vi "Drive Controller.vi"(8 "error in":errorcluster) -> ()   [LabVIEW 2019]
doc: "This VI executes continuously carrying out the current operation and responding to updates or new operation requests. It will often contain the timing or control code that is difficult to place directly in TeleOp. This VI generally opens all sensors and motors and isolates the rest of the robot code from knowing implementation details of how the operations are carried out."
uses:
  <vilib>/Rock Robotics/WPI/Framework/Completion Status.ctl
  Drive Setpoints.ctl
  Drive Operations.ctl
  <vilib>/Rock Robotics/WPI/ThirdParty/REV Robotics/SPARK MAX/Typedef/Spark MAX Control Type.ctl
panel:
  out "L v 2":dbl(graph)
  out "L setpoint 2":dbl(graph)
  out "R setpoint 2":dbl(graph)
  out "R v":dbl(graph)
  out "L v":dbl(graph)
  out "L setpoint":dbl(graph)
  out "R setpoint":dbl(graph)
  out "Immediate graph":dbl(graph)
  in  "Interactive Values":T1
  in  "Buttons":cluster{"Execute Cmd":bool, "Abort Cmd":bool}
  out "Command Timing":cluster{"Start Time (ms)":u32, "Iterations":i32}
  out "Status":T3
  out "Current\nCmd":string
  # "Tip: The graph shows the motor setpoints. It may also be helpful to observe inputs and sensor values.\nYou may also want to display tuning or debugging controls."
  # "Interactive Command: You may fill in the settings for a command\nand schedule it with the Execute button. You can observe and abort\nany command while fine tuning the code for the controller."
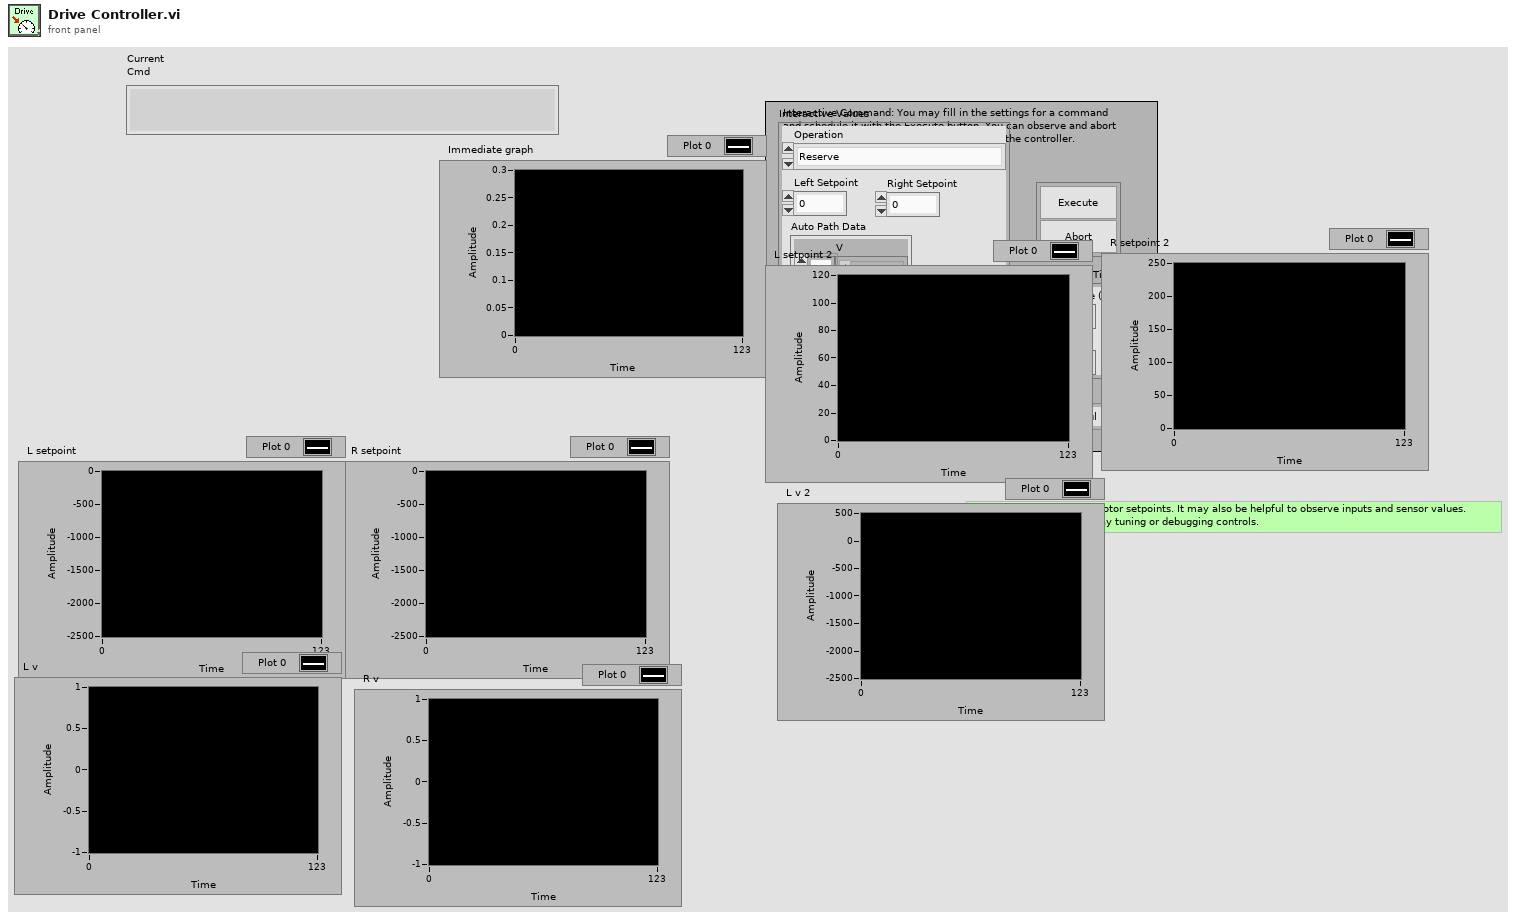
[diagram p1: front panel]
types:
  T1 = typedef "Drive Setpoints.ctl" = cluster{"Operation":T2, "Left Setpoint":dbl, "Right Setpoint":dbl, "Auto Path Data":cluster{"V":dbl[], "Theta":dbl[], "Sample Period":dbl}}
  T2 = typedef "Drive Operations.ctl" = enum16{"Reserve", "Read Current", "Immediate", "Drive for Time", "Drive for Distance", "Play Path", "Play Path Rev"}
  T3 = typedef "Completion Status.ctl" = enum16{"Successful", "Aborted", "Incomplete"}
  T4 = typedef "WPI_MotorControlDeviceRef.ctl" = cluster{"DeviceStatus":errorcluster, "Type":T5, "PWM":cluster{"PWM Channel":T6, "DeadBand":T7}, "CAN":cluster{"Device Number":u8, "SetOutput VI Ref":variant, "GetOutput VI Ref":variant, "Enable VI Ref":variant, "Disable VI Ref":variant, "Data":variant}, "Invert":bool, "DIO PWM":cluster{"PWM \"Enable\" Channel":T6, "DIOChannel":T8, "PWM Rate":dbl}}
  T5 = typedef "WPI_MotorControlType.ctl" = enum16{"PWM", "CAN", "DIO PWM"}
  T6 = typedef "FPGA_DIOPWMChannel.ctl" = enum8{"PWM 0", "PWM 1", "PWM 2", "PWM 3", "PWM 4", "PWM 5", "PWM 6", "PWM 7", "PWM 8", "PWM 9", "PWM MXP 0", "PWM MXP 1", "PWM MXP 2", "PWM MXP 3", "PWM MXP 4", "PWM MXP 5", "PWM MXP 6", "PWM MXP 7", "PWM MXP 8", "PWM MXP 9", "Invalid"}
  T7 = typedef "WPI_PWMDeadband.ctl" = cluster{"Name":string, "maxPositivePwm":i32, "minPositivePwm":i32, "centerPwm":i32, "maxNegativePwm":i32, "minNegativePwm":i32, "angularRange":u16}
  T8 = typedef "FPGA_DIOChannel.ctl" = enum8{"DIO 0", "DIO 1", "DIO 2", "DIO 3", "DIO 4", "DIO 5", "DIO 6", "DIO 7", "DIO 8", "DIO 9", "DIO MXP 0", "DIO MXP 1", "DIO MXP 2", "DIO MXP 3", "DIO MXP 4", "DIO MXP 5", "DIO MXP 6", "DIO MXP 7", "DIO MXP 8", "DIO MXP 9", "DIO MXP 10", "DIO MXP 11", "DIO MXP 12", "DIO MXP 13", "DIO MXP 14", "DIO MXP 15", "SPI Port CS1", "SPI Port CS2", "SPI Port CS3", "SPI Port MISO", "SPI Port MOSI", "Invalid"}
  T9 = typedef "Command Status Info.ctl" = cluster{"Name":string, "Status":T3, "notifier out":T10}
  T10 = typedef "Completion Notifier.ctl" = refnum<notifier>
  T11 = cluster{"SubSystem Data":T1, cluster{"Start Time (ms)":u32, "Iterations":i32}, cluster{"Command Info":T9, "Description":string, "Default Command":T1, "queue out":refnum<queue>, "Subsystem Name":string}}
  T12 = typedef "Spark MAX Control Type.ctl" = enum16{"Percent VBus", "Voltage", "Velocity", "Position", "Smart Motion", "Current", "Smart Velocity"}
  T13 = cluster{"V":dbl[], "Theta":dbl[], "Sample Period":dbl}
  T14 = cluster{"SubSystem Data":T1, cluster{"Start Time (ms)":u32, "Iterations":i32}, "Default Command Arguments":cluster{"Command Info":T9, "Description":string, "Default Command":T1, "queue out":refnum<queue>, "Subsystem Name":string}}
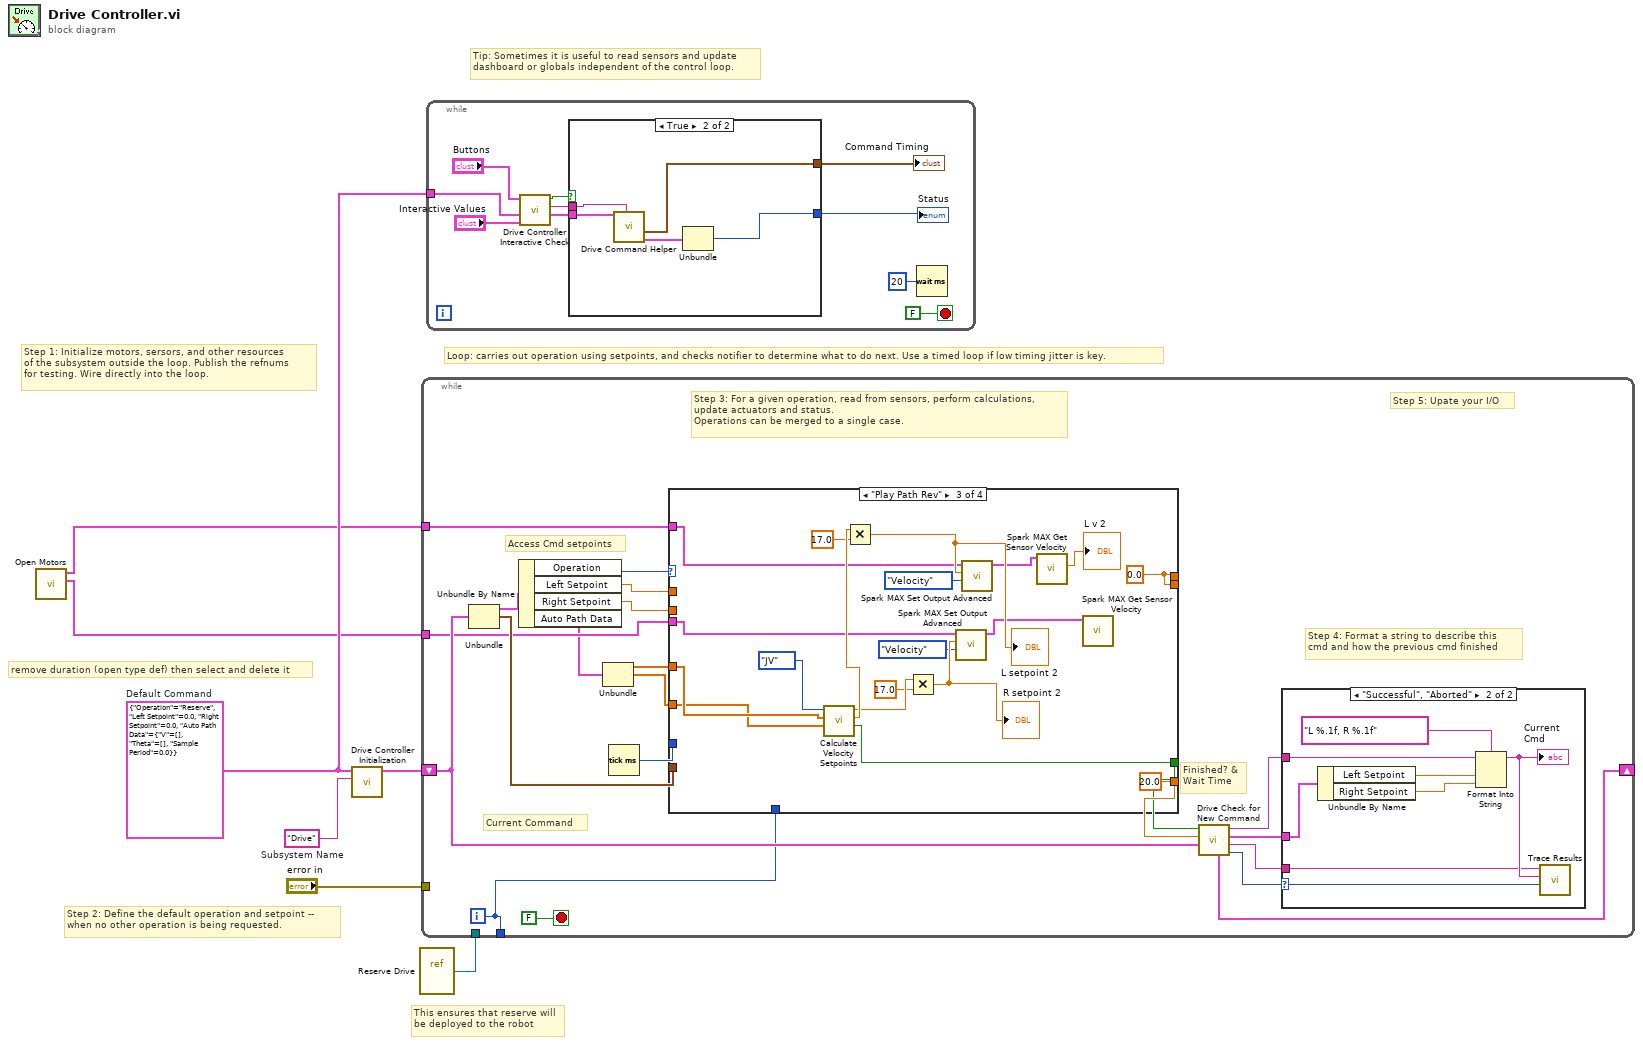
[diagram p0: block diagram]
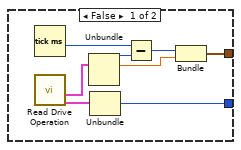
[diagram p2: hidden frame]
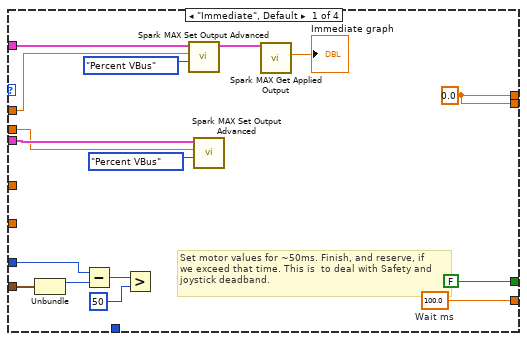
[diagram p4: hidden frame]
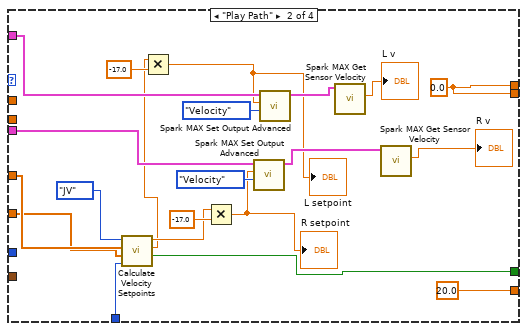
[diagram p5: hidden frame]
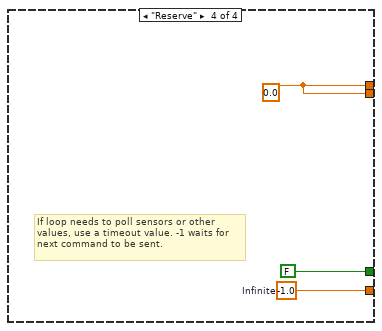
[diagram p6: hidden frame]
diagram:
  w3 = T1 {"Operation"=enum."Reserve", "Left Setpoint"=0.0, "Right Setpoint"=0.0, "Auto Path Data"={"V"=[], "Theta"=[], "Sample Period"=0.0}}  # Default Command
  w7 = "Drive"  # Subsystem Name
  # "remove duration (open type def) then select and delete it"
  # "This ensures that reserve will\nbe deployed to the robot"
  # "Tip: Sometimes it is useful to read sensors and update\ndashboard or globals independent of the control loop."
  # "Step 2: Define the default operation and setpoint --\nwhen no other operation is being requested."
  # "Step 1: Initialize motors, sersors, and other resources\nof the subsystem outside the loop. Publish the refnums\nfor testing. Wire directly into the loop."
  # "Loop: carries out operation using setpoints, and checks notifier to determine what to do next. Use a timed loop if low timing jitter is key."
  n1 = call "Open Motors.vi"() -> ("Right"=w1:T4, "Left"=w2:T4)  [unwired: 10 in]
  n2 = call "Drive Controller Initialization.vi"("Subsystem Name"=w7, "Default Command"=w3) -> ("Current Command"=w5:T11)  [unwired: 9 in]
  n3 = vi-ref "Reserve Drive.vi"() -> (w4:refnum<vi>)
  n4 = while {
    shift-right: [w21] -> _
    shift-left: w5 -> [w14]
    tunnel: [w8] -> _
    tunnel: "error in" -> [_]
    tunnel: w4 -> [_]
    tunnel: w2 -> [w13]
    tunnel: w1 -> [w12]
    i -> [w8]
    stop <- FALSE stop-if-true
    # "Step 5: Upate your I/O"
    # "Step 4: Format a string to describe this\ncmd and how the previous cmd finished"
    # "Current Command"
    # "Access Cmd setpoints"
    # "Finished? &\nWait Time"
    # "Step 3: For a given operation, read from sensors, perform calculations,\nupdate actuators and status.\nOperations can be merged to a single case."
    n5 = Unbundle(w14) -> ("SubSystem Data"=w27:T1, w15:cluster{"Start Time (ms)":u32, "Iterations":i32})  [unwired: 1 out]
    n6 = Unbundle By Name(w27) -> ("Operation"=w26:T2, "Left Setpoint"=w25:dbl, "Right Setpoint"=w24:dbl, "Auto Path Data"=w11:T13)
    n7 = Unbundle(w11) -> ("V"=w10:dbl[], "Theta"=w9:dbl[])  [unwired: 1 out]
    n8 = Tick Count (ms)() -> (millisecond timer value=w23:u32)
    n9 = case shown="\"Play Path Rev\"" w26 {
      tunnel: [w52 20.0 ("Infinite") 20.0 ("Infinite") w95] -> w20
      tunnel: [FALSE ("ignore previous (F)") w63 w75 FALSE ("ignore previous (F)")] -> w19
      tunnel: w15 -> [w47 _ _ _]
      tunnel: [w39 w73 w76 w93] -> _
      tunnel: [w39 w73 w76 w93] -> _
      tunnel: w25 -> [w43 _ _ _]
      tunnel: w24 -> [w40 _ _ _]
      tunnel: w23 -> [w48 _ _ _]
      tunnel: w13 -> [w45 w72 w80 _]
      tunnel: w12 -> [w41 w71 w79 _]
      tunnel: w10 -> [_ w66 w78 _]
      tunnel: w9 -> [_ w65 w77 _]
      tunnel: w8 -> [_ w64 _ _]
      frame "Immediate", Default {
        w39 = 0.0
        w52 = 100.0  # Wait ms
        # "Set motor values for ~50ms. Finish, and reserve, if\nwe exceed that time. This is  to deal with Safety and\njoystick deadband."
        n10 = Unbundle(w47) -> ("Start Time (ms)"=w49:u32)  [unwired: 1 out]
        n11 = Subtract(x=w48, y=w49) -> (x-y=w50:u32)
        n12 = Greater?(x=w50, y=u8 50 ("Left Motor")) -> ()  [unwired: 1 out]
        n13 = call <vilib>:"Spark MAX Set Output Advanced.vi"("Control Mode"=Spark_MAX_Control_Type."Percent VBus", "Setpoint"=w43, "MotorControlDevRef"=w45) -> ("MotorControlDevRef"=w38:T4)  [unwired: 7 in, 1 out]
        n14 = call <vilib>:"Spark MAX Set Output Advanced.vi"("Control Mode"=Spark_MAX_Control_Type."Percent VBus", "Setpoint"=w40, "MotorControlDevRef"=w41) -> ()  [unwired: 7 in, 2 out]
        n15 = call <vilib>:"Spark MAX Get Applied Output.vi"("MotorControlDevRef in"=w38) -> ("Applied Output"=→"Immediate graph":dbl)  [unwired: 7 in, 3 out]
      }
      frame "Play Path" {
        w73 = 0.0
        n16 = call "Calculate Velocity Setpoints.vi"("Iterations"=w64, "Angular Data (Relative)"=w65, "Velocity Data"=w66, "Enum"=enum16{"JV", "Mule", "Linda/Sophie"}."JV") -> ("Finished?"=w63:bool, "Right Setpoint"=w59:dbl, "Left Setpoint"=w60:dbl)  [unwired: 5 in]
        n17 = Multiply(x=w59, y=-17.0) -> (x*y=w54:dbl)
        "L setpoint" <- w54
        n18 = Multiply(x=w60, y=-17.0) -> (x*y=w53:dbl)
        "R setpoint" <- w53
        n19 = call <vilib>:"Spark MAX Set Output Advanced.vi"("Control Mode"=Spark_MAX_Control_Type."Velocity", "Setpoint"=w53, "MotorControlDevRef"=w71) -> ("MotorControlDevRef"=w57:T4)  [unwired: 7 in, 1 out]
        n20 = call <vilib>:"Spark MAX Set Output Advanced.vi"("Control Mode"=Spark_MAX_Control_Type."Velocity", "Setpoint"=w54, "MotorControlDevRef"=w72) -> ("MotorControlDevRef"=w58:T4)  [unwired: 7 in, 1 out]
        n21 = call <vilib>:"Spark MAX Get Sensor Velocity.vi"("MotorControlDevRef in"=w58) -> ("Sensor Velocity"=→"L v":dbl)  [unwired: 7 in, 3 out]
        n22 = call <vilib>:"Spark MAX Get Sensor Velocity.vi"("MotorControlDevRef in"=w57) -> ("Sensor Velocity"=→"R v":dbl)  [unwired: 7 in, 3 out]
      }
      frame "Play Path Rev" {
        w76 = 0.0
        n23 = call "Calculate Velocity Setpoints.vi"("Angular Data (Relative)"=w77, "Velocity Data"=w78, "Enum"=enum16{"JV", "Mule", "Linda/Sophie"}."JV") -> ("Finished?"=w75:bool, "Right Setpoint"=w87:dbl, "Left Setpoint"=w86:dbl)  [unwired: 6 in]
        n24 = Multiply(x=w87, y=17.0) -> (x*y=w91:dbl)
        "L setpoint 2" <- w91
        n25 = Multiply(x=w86, y=17.0) -> (x*y=w92:dbl)
        "R setpoint 2" <- w92
        n26 = call <vilib>:"Spark MAX Set Output Advanced.vi"("Control Mode"=Spark_MAX_Control_Type."Velocity", "Setpoint"=w92, "MotorControlDevRef"=w79) -> ("MotorControlDevRef"=w89:T4)  [unwired: 7 in, 1 out]
        n27 = call <vilib>:"Spark MAX Set Output Advanced.vi"("Control Mode"=Spark_MAX_Control_Type."Velocity", "Setpoint"=w91, "MotorControlDevRef"=w80) -> ("MotorControlDevRef"=w88:T4)  [unwired: 7 in, 1 out]
        n28 = call <vilib>:"Spark MAX Get Sensor Velocity.vi"("MotorControlDevRef in"=w88) -> ("Sensor Velocity"=→"L v 2":dbl)  [unwired: 7 in, 3 out]
        n29 = call <vilib>:"Spark MAX Get Sensor Velocity.vi"("MotorControlDevRef in"=w89) -> ()  [unwired: 7 in, 4 out]
      }
      frame "Reserve" {
        w93 = 0.0
        w95 = -1.0  # Infinite
        # "If loop needs to poll sensors or other\nvalues, use a timeout value. -1 waits for\nnext command to be sent."
      }
    }
    n30 = call "Drive Check for New Command.vi"("input cluster"=w14, "Wait time (ms)"=w20, "Finished?"=w19) -> ("Completion"=w22:T3, "Subsystem Name"=w16:string, "Current Command"=w17:T1, "Initial Trace String"=w18:string, "Next Command"=w21:T14)  [unwired: 4 in]
    n31 = case shown="\"Successful\", \"Aborted\"" w22 {
      selector: w22 -> [_ w36]
      tunnel: w18 -> [_ w31]
      tunnel: w17 -> [_ w32]
      tunnel: w16 -> [_ w29]
      frame "Incomplete", Default {
        # "Continuing current command"
      }
      frame "Successful", "Aborted" {
        # "Report and setup for next command"
        n32 = Unbundle By Name(w32) -> ("Left Setpoint"=w34:dbl, "Right Setpoint"=w35:dbl)
        n33 = Format Into String(format string="L %.1f, R %.1f", initial string=w31, w34, w35) -> (resulting string=w30:string)  [unwired: 1 in, 1 out]
        "Current\nCmd" <- w30
        n34 = call <vilib>:"Trace Results.vi"("Status of previous command"=w36, "Description"=w30, "Subsystem"=w29) -> ()  [unwired: 9 in]
      }
    }
  }
  n35 = while {
    tunnel: w3 -> [w97]
    stop <- FALSE stop-if-true
    n36 = call "Drive Controller Interactive Check.vi"("Interactive Command In"="Interactive Values", "Default Command"=w97, "Buttons"="Buttons") -> ("Interactive Command Out"=w99:T1, "Trace String"=w100:string, "Schedule"=w101:bool)  [unwired: 6 in]
    n37 = case shown="True" w101 {
      tunnel: [w110 w118] -> w102
      tunnel: [w109 w114] -> w103
      tunnel: w100 -> [_ w116]
      tunnel: w99 -> [_ w115]
      frame False {
        n38 = Tick Count (ms)() -> (millisecond timer value=w113:u32)
        n39 = call "Read Drive Operation.vi"() -> ("Command Info"=w107:T9, "SubSystem Data"=w106:T1)  [unwired: 9 in, 1 out]
        n40 = Unbundle(w106) -> ("Operation"=w111:T2, "Left Setpoint"=w108:dbl)  [unwired: 2 out]
        n41 = Unbundle(w107) -> ("Status"=w110:T3)  [unwired: 2 out]
        n42 = Subtract(x=w113, y=w111) -> (x-y=w112:u32)
        n43 = Bundle(w112, "Left Setpoint"=w108) -> (w109:cluster{u32, "Left Setpoint":dbl})  [unwired: 1 in]
      }
      frame True {
        n44 = call "Drive Command Helper.vi"("Description"=w116, "SubSystem Data"=w115) -> ("Command Info Out"=w117:T9, "Command Timing"=w114:cluster{"Start Time (ms)":u32, "Iterations":i32})  [unwired: 7 in, 1 out]
        n45 = Unbundle(w117) -> ("Status"=w118:T3)  [unwired: 2 out]
      }
    }
    "Status" <- w102
    "Command Timing" <- w103
    n46 = Wait (ms)(milliseconds to wait=u32 20) -> ()  [unwired: 1 out]
  }
